vi "SetDOOutPut.vi"(8 "错误输入（无错误）":errorcluster) -> (0 "错误输出":errorcluster)   [LabVIEW 2014]
uses:
  X86Dll/ZXUTConfigMgr.dll
panel:
  in  "输出值":u8
  in  "管脚序号":u8
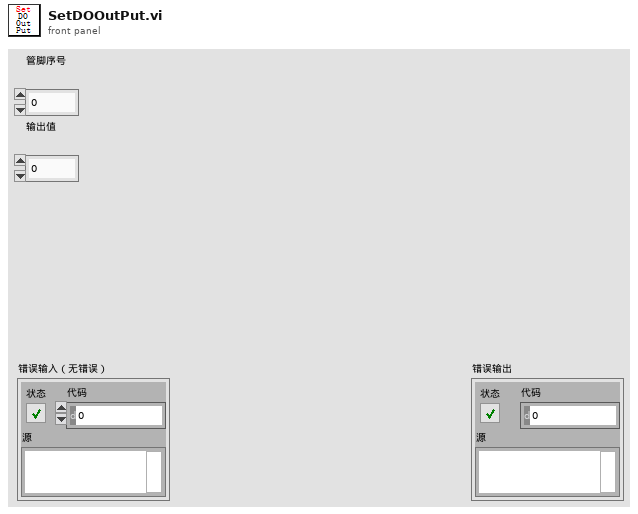
[diagram p1: front panel]
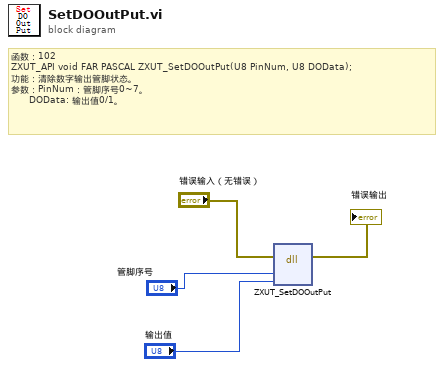
[diagram p0: block diagram]
diagram:
  # "函数：102\nZXUT_API void\tFAR PASCAL ZXUT_SetDOOutPut(U8 PinNum, U8 DOData);\n功能：清除数字输出管脚状态。\n参数：PinNum：管脚序号0~7。\n      DOData: 输出值0/1。"
  n1 = dll-call lib="D:/Software/Utrasonic on-line monitoring/X86Dll/ZXUTConfigMgr.dll" fn="ZXUT_SetDOOutPut"(error in="错误输入（无错误）", "PinNum"="管脚序号", "DOData"="输出值") -> (error out=→"错误输出":errorcluster)  [unwired: 5 in, 1 out]
